vi "Send CMD_M1.vi"(5 "Speed (mm/s) M1":i32, 6 "SERVO ON CMD M1":bool, 8 "Home Calling M1":bool, 9 "Pokayoka":bool, 10 "Travel (mm)M1":i32, 11 "Slide Servo":T1) -> ()   [LabVIEW 2015]
uses:
  Galobal variable_TI.vi
  Project Setup/Globle Variable/GR_Servo.vi
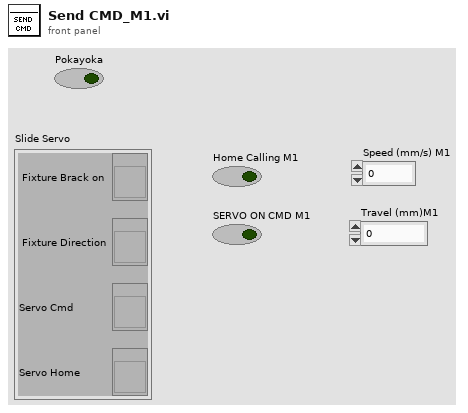
[diagram p1: front panel]
types:
  T1 = cluster{" Fixture Brack on":refnum<vi>, " Fixture Direction":refnum<vi>, "Servo Cmd":refnum<vi>, "Servo Home":refnum<vi>}
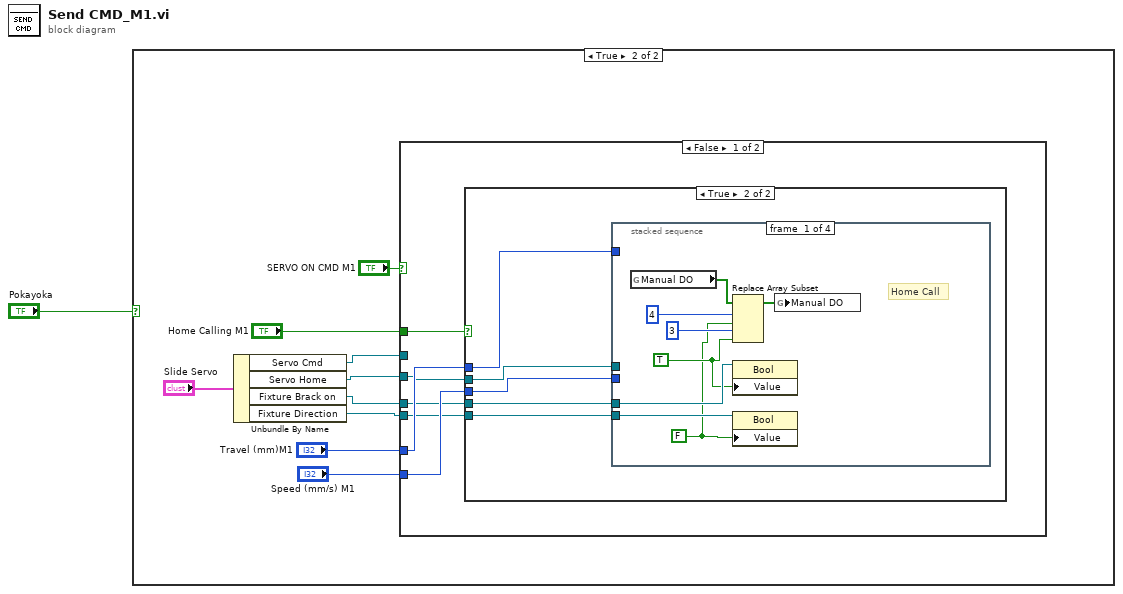
[diagram p0: block diagram]
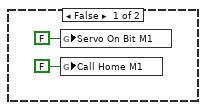
[diagram p3: hidden frame]
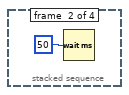
[diagram p4: hidden frame]
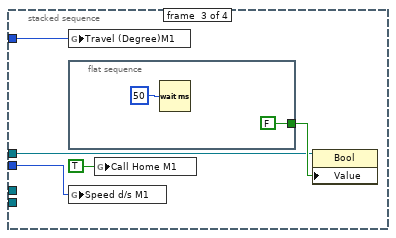
[diagram p5: hidden frame]
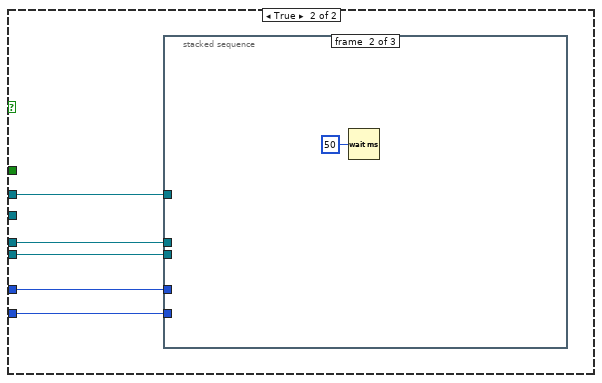
[diagram p7: hidden frame]
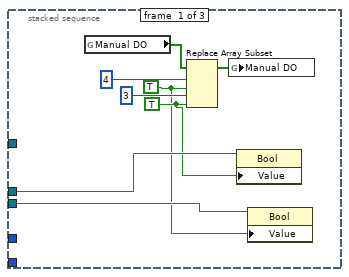
[diagram p8: hidden frame]
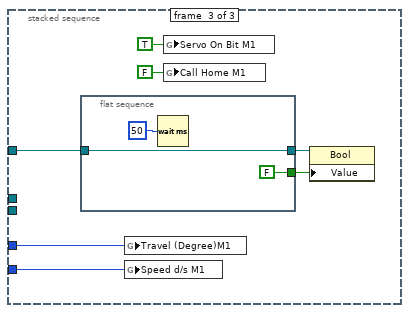
[diagram p9: hidden frame]
diagram:
  n1 = case shown="True" "Pokayoka" {
    frame False {
    }
    frame True {
      n2 = Unbundle By Name("Slide Servo") -> ("Servo Cmd"=w2:refnum<vi>, "Servo Home"=w3:refnum<vi>, "Fixture Brack on"=w5:refnum<vi>, "Fixture Direction"=w4:refnum<vi>)
      n3 = case shown="False" "SERVO ON CMD M1" {
        tunnel: "Speed (mm/s) M1" -> [w15 w44]
        tunnel: "Travel (mm)M1" -> [w14 w43]
        tunnel: "Home Calling M1" -> [w16 _]
        tunnel: w2 -> [_ w42]
        tunnel: w3 -> [w13 _]
        tunnel: w5 -> [w12 w41]
        tunnel: w4 -> [w11 w40]
        frame False {
          n4 = case shown="True" w16 {
            tunnel: w15 -> [_ w20]
            tunnel: w14 -> [_ w19]
            tunnel: w13 -> [_ w21]
            tunnel: w12 -> [_ w23]
            tunnel: w11 -> [_ w22]
            frame False {
              n5 = global write "GR_Servo.vi" "Servo On Bit M1"(FALSE ("Servo On Bit")) -> ()
              n6 = global write "Galobal variable_TI.vi" "Call Home M1"(FALSE ("Call Home M1")) -> ()
            }
            frame True {
              n7 = stacked-sequence {
                tunnel: w23 -> [w29 _ _ _]
                tunnel: w22 -> [w28 _ _ _]
                tunnel: w21 -> [_ _ w35 _]
                tunnel: w20 -> [_ _ w34 _]
                tunnel: w19 -> [_ _ w33 _]
                frame #0 {
                  w25 = TRUE ("new element/subarray")
                  w24 = FALSE ("new element/subarray")
                  # "Home Call"
                  n8 = global read "Galobal variable_TI.vi" "Manual DO"() -> (w26:bool[])
                  n9 = Replace Array Subset(array=w26, new element #1=w24, index #1=4 ("index"), new element #2=w25, index #2=3 ("index")) -> (w31:bool[])
                  n10 = property class="Bool"(reference=w29, "Value"=w25) -> ()  [unwired: 1 in, 2 out]
                  n11 = property class="Bool"(reference=w28, "Value"=w24) -> ()  [unwired: 1 in, 2 out]
                  n12 = global write "Galobal variable_TI.vi" "Manual DO"(w31) -> ()
                }
                frame #1 {
                  n13 = Wait (ms)(milliseconds to wait=u32 50) -> ()  [unwired: 1 out]
                }
                frame #2 {
                  n14 = global write "GR_Servo.vi" "Travel (Degree)M1"(w33) -> ()
                  n15 = flat-sequence {
                    tunnel: [FALSE ("SERVO ON CMD M1")] -> w36
                    frame #0 {
                      n16 = Wait (ms)(milliseconds to wait=u32 50) -> ()  [unwired: 1 out]
                    }
                  }
                  n17 = global write "GR_Servo.vi" "Speed d/s M1"(w34) -> ()
                  n18 = global write "Galobal variable_TI.vi" "Call Home M1"(TRUE ("Call Home M1")) -> ()
                  n19 = property class="Bool"(reference=w35, "Value"=w36) -> ()  [unwired: 1 in, 2 out]
                }
                frame #3 {
                }
              }
            }
          }
        }
        frame True {
          n20 = stacked-sequence {
            tunnel: w44 -> [_ _ w60]
            tunnel: w43 -> [_ _ w59]
            tunnel: w42 -> [_ _ w56]
            tunnel: w41 -> [w48 _ _]
            tunnel: w40 -> [w47 _ _]
            frame #0 {
              w46 = TRUE ("new element/subarray")
              w45 = TRUE ("new element/subarray")
              n21 = global read "Galobal variable_TI.vi" "Manual DO"() -> (w49:bool[])
              n22 = Replace Array Subset(array=w49, new element #1=w45, index #1=4 ("index"), new element #2=w46, index #2=3 ("index")) -> (w52:bool[])
              n23 = global write "Galobal variable_TI.vi" "Manual DO"(w52) -> ()
              n24 = property class="Bool"(reference=w48, "Value"=w46) -> ()  [unwired: 1 in, 2 out]
              n25 = property class="Bool"(reference=w47, "Value"=w45) -> ()  [unwired: 1 in, 2 out]
            }
            frame #1 {
              n26 = Wait (ms)(milliseconds to wait=u32 50) -> ()  [unwired: 1 out]
            }
            frame #2 {
              n27 = flat-sequence {
                tunnel: [w62] -> w55
                tunnel: w56 -> [w62]
                tunnel: [FALSE ("SERVO ON CMD M1")] -> w54
                frame #0 {
                  n28 = Wait (ms)(milliseconds to wait=u32 50) -> ()  [unwired: 1 out]
                }
              }
              n29 = global write "GR_Servo.vi" "Travel (Degree)M1"(w59) -> ()
              n30 = global write "GR_Servo.vi" "Speed d/s M1"(w60) -> ()
              n31 = global write "GR_Servo.vi" "Servo On Bit M1"(TRUE ("Servo On Bit")) -> ()
              n32 = global write "Galobal variable_TI.vi" "Call Home M1"(FALSE ("Call Home M1")) -> ()
              n33 = property class="Bool"(reference=w55, "Value"=w54) -> ()  [unwired: 1 in, 2 out]
            }
          }
        }
      }
    }
  }
